vi "Rename Configuration LLB in LVPROJ.vi"(8 "error in":errorcluster, 9 "CD lvproj name":string, 10 "CD name":string, 11 "custom device path":path) -> (0 "error out":errorcluster, 3 "custom device path out":path)   [LabVIEW 2020, in "Template Tool.lvlib"]
uses:
  Template Tool.lvlib
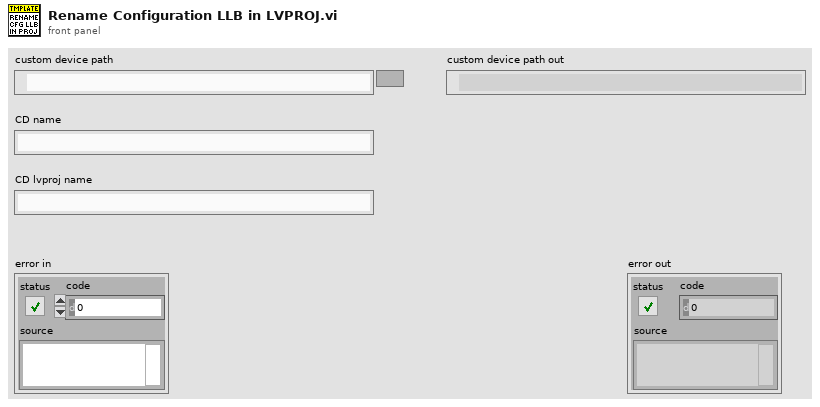
[diagram p1: front panel]
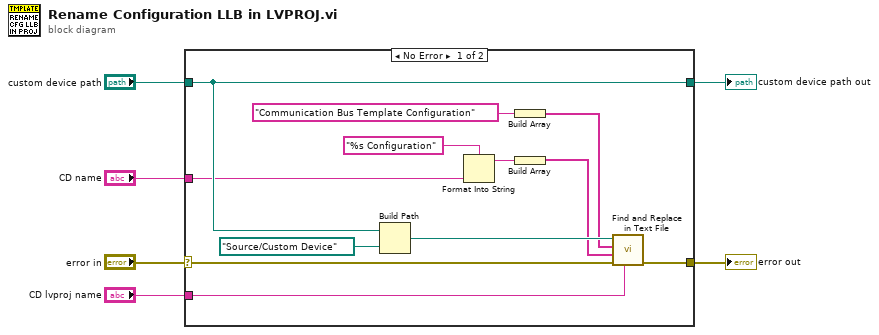
[diagram p0: block diagram]
diagram:
  n1 = case shown="No Error" "error in" {
    selector: "error in" -> [w17 w19]
    tunnel: "custom device path" -> [w16 w20]
    tunnel: [w15 w19] -> w6
    tunnel: [w16 w20] -> w3
    tunnel: "CD name" -> [w8 _]
    tunnel: "CD lvproj name" -> [w7 _]
    frame No Error {
      n2 = Build Path(base path=w16, name or relative path=path "Source/Custom Device") -> (appended path=w14:path)
      n3 = Format Into String(format string="%s Configuration" ("string"), w8) -> (resulting string=w9:string)  [unwired: 2 in, 1 out]
      n4 = Build Array("Communication Bus Template Configuration" ("string")) -> (w12:string[])
      n5 = Build Array(w9) -> (w11:string[])
      n6 = call "Find and Replace in Text File.vi"("file name"=w7, "error in"=w17, "replace array"=w11, "find array"=w12, "folder path"=w14) -> ("error out"=w15:errorcluster)  [unwired: 5 in, 1 out]
    }
    frame Error {
    }
  }
  "error out" <- w6
  "custom device path out" <- w3
